vi "addViToLib.vi"(8 "error in (no error)":errorcluster, 10 "arrayOfVi":path[](array[path]), 11 "libRefIn":refnum<vi>) -> (0 "error out":errorcluster, 3 "libRefOut":refnum<vi>)   [LabVIEW 2018]
doc: "Add the vi to LabVIEW library."
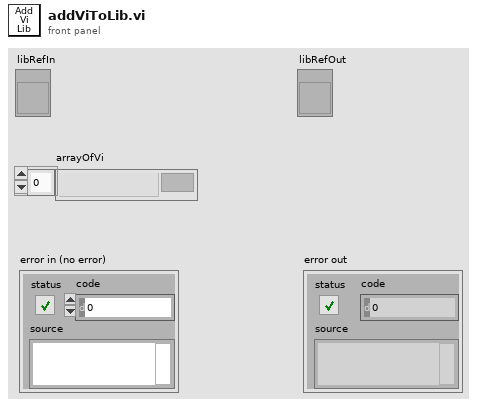
[diagram p1: front panel]
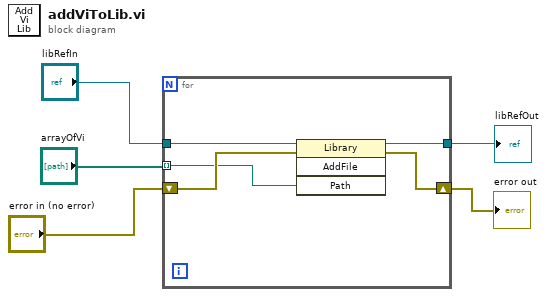
[diagram p0: block diagram]
diagram:
  n1 = for {
    shift-right: [w6] -> w1
    shift-left: "error in (no error)" -> [w9]
    tunnel: "libRefIn" -> [w10]
    tunnel: [w8] -> w2
    tunnel: "arrayOfVi" -> [w7] mode=indexing
    n2 = invoke class="Library" method="AddFile"(reference=w10, error in=w9, "Path"=w7) -> (reference out=w8:refnum<vi>, error out=w6:errorcluster)  [unwired: 1 in, 2 out]
  }
  "error out" <- w1
  "libRefOut" <- w2
